vi "GEA2 Serial Send Command.vi"(6 "Retry":i32=3, 8 "error in (no error)":errorcluster, 9 "Byte Count":u32, 10 "Message Out":u8[](array[numeric]), 11 "VISA Refnum in":refnum<visa-resource-name>) -> (0 "error out":errorcluster, 3 "WriteOK":bool)   [LabVIEW 2014]
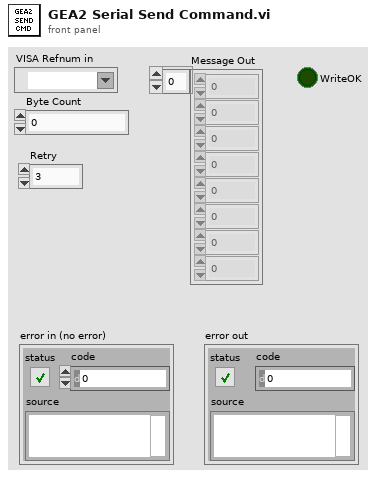
[diagram p1: front panel]
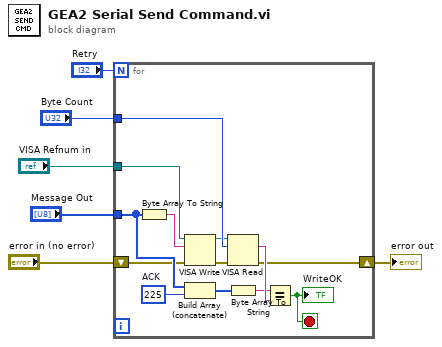
[diagram p0: block diagram]
diagram:
  n1 = for {
    N: "Retry" -> [_]
    tunnel: "Byte Count" -> [w19]
    tunnel: "Message Out" -> [w17]
    tunnel: "VISA Refnum in" -> [w8]
    shift-right: [w13] -> w4
    shift-left: "error in (no error)" -> [w12]
    stop <- w7 stop-if-true
    w14 = u8 225  # ACK
    n2 = Byte Array To String(unsigned byte array=w17) -> (string=w16:string)
    n3 = VISA Write(VISA resource name=w8, write buffer=w16, error in (no error)=w12) -> (VISA resource name out=w9:refnum<visa-resource-name>, error out=w10:errorcluster)  [unwired: 1 out]
    n4 = Build Array (concatenate)(w17, w14) -> (w15:u8[])
    n5 = VISA Read(VISA resource name=w9, byte count=w19, error in (no error)=w10) -> (read buffer=w18:string, error out=w13:errorcluster)  [unwired: 2 out]
    n6 = Byte Array To String(unsigned byte array=w15) -> (string=w11:string)
    n7 = Equal?(x=w11, y=w18) -> (x = y?=w7:bool)
    "WriteOK" <- w7
  }
  "error out" <- w4
